vi "subscribeCommands.vi"(8 "error in (no error)":errorcluster, 11 "SAL_Listener in":refnum<class "SAL_Listener.lvclass">) -> (0 "error out":errorcluster, 3 "SAL_Listener out":refnum<class "SAL_Listener.lvclass">)   [LabVIEW 2016, in "SAL_Listener.lvclass"]
uses:
  SAL_Listener.lvclass
  SALLV_dome/SALLV_dome.lvlib
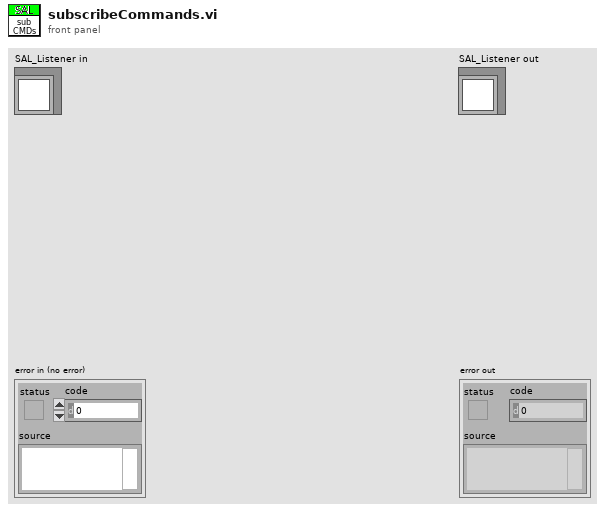
[diagram p1: front panel]
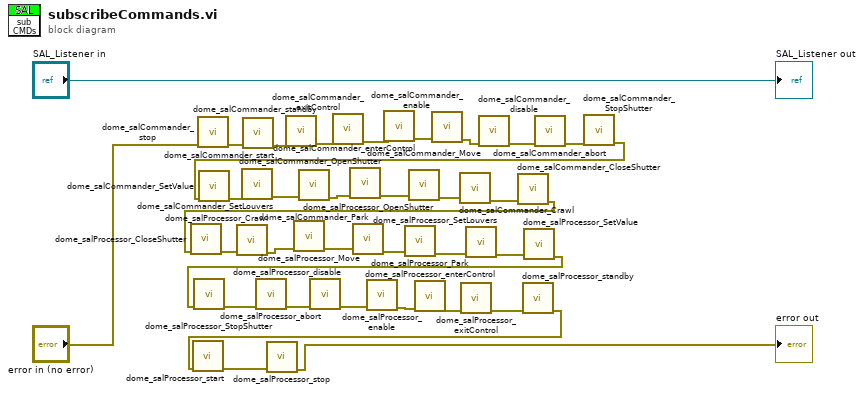
[diagram p0: block diagram]
diagram:
  n1 = call "dome_salCommander_stop.vi"("error in (no error)"="error in (no error)") -> ("error out"=w32:errorcluster)  [unwired: 9 in, 1 out]
  n2 = call "dome_salCommander_start.vi"("error in (no error)"=w32) -> ("error out"=w31:errorcluster)  [unwired: 9 in, 1 out]
  n3 = call "dome_salCommander_standby.vi"("error in (no error)"=w31) -> ("error out"=w30:errorcluster)  [unwired: 9 in, 1 out]
  n4 = call "dome_salCommander_exitControl.vi"("error in (no error)"=w30) -> ("error out"=w29:errorcluster)  [unwired: 9 in, 1 out]
  n5 = call "dome_salCommander_enterControl.vi"("error in (no error)"=w29) -> ("error out"=w28:errorcluster)  [unwired: 9 in, 1 out]
  n6 = call "dome_salCommander_enable.vi"("error in (no error)"=w28) -> ("error out"=w27:errorcluster)  [unwired: 9 in, 1 out]
  n7 = call "dome_salCommander_disable.vi"("error in (no error)"=w27) -> ("error out"=w26:errorcluster)  [unwired: 9 in, 1 out]
  n8 = call "dome_salCommander_abort.vi"("error in (no error)"=w26) -> ("error out"=w24:errorcluster)  [unwired: 9 in, 1 out]
  n9 = call "dome_salCommander_StopShutter.vi"("error in (no error)"=w24) -> ("error out"=w25:errorcluster)  [unwired: 9 in, 1 out]
  n10 = call "dome_salCommander_SetValue.vi"("error in (no error)"=w25) -> ("error out"=w23:errorcluster)  [unwired: 9 in, 1 out]
  n11 = call "dome_salCommander_SetLouvers.vi"("error in (no error)"=w23) -> ("error out"=w22:errorcluster)  [unwired: 9 in, 1 out]
  n12 = call "dome_salCommander_Park.vi"("error in (no error)"=w22) -> ("error out"=w21:errorcluster)  [unwired: 9 in, 1 out]
  n13 = call "dome_salCommander_OpenShutter.vi"("error in (no error)"=w21) -> ("error out"=w20:errorcluster)  [unwired: 9 in, 1 out]
  n14 = call "dome_salCommander_Move.vi"("error in (no error)"=w20) -> ("error out"=w19:errorcluster)  [unwired: 9 in, 1 out]
  n15 = call "dome_salCommander_Crawl.vi"("error in (no error)"=w19) -> ("error out"=w18:errorcluster)  [unwired: 9 in, 1 out]
  n16 = call "dome_salCommander_CloseShutter.vi"("error in (no error)"=w18) -> ("error out"=w17:errorcluster)  [unwired: 9 in, 1 out]
  n17 = call "dome_salProcessor_CloseShutter.vi"("error in (no error)"=w17) -> ("error out"=w16:errorcluster)  [unwired: 9 in, 1 out]
  n18 = call "dome_salProcessor_Crawl.vi"("error in (no error)"=w16) -> ("error out"=w15:errorcluster)  [unwired: 9 in, 1 out]
  n19 = call "dome_salProcessor_Move.vi"("error in (no error)"=w15) -> ("error out"=w14:errorcluster)  [unwired: 9 in, 1 out]
  n20 = call "dome_salProcessor_OpenShutter.vi"("error in (no error)"=w14) -> ("error out"=w13:errorcluster)  [unwired: 9 in, 1 out]
  n21 = call "dome_salProcessor_Park.vi"("error in (no error)"=w13) -> ("error out"=w12:errorcluster)  [unwired: 9 in, 1 out]
  n22 = call "dome_salProcessor_SetLouvers.vi"("error in (no error)"=w12) -> ("error out"=w11:errorcluster)  [unwired: 9 in, 1 out]
  n23 = call "dome_salProcessor_SetValue.vi"("error in (no error)"=w11) -> ("error out"=w10:errorcluster)  [unwired: 9 in, 1 out]
  n24 = call "dome_salProcessor_StopShutter.vi"("error in (no error)"=w10) -> ("error out"=w9:errorcluster)  [unwired: 9 in, 1 out]
  n25 = call "dome_salProcessor_abort.vi"("error in (no error)"=w9) -> ("error out"=w8:errorcluster)  [unwired: 9 in, 1 out]
  n26 = call "dome_salProcessor_disable.vi"("error in (no error)"=w8) -> ("error out"=w7:errorcluster)  [unwired: 9 in, 1 out]
  n27 = call "dome_salProcessor_enable.vi"("error in (no error)"=w7) -> ("error out"=w6:errorcluster)  [unwired: 9 in, 1 out]
  n28 = call "dome_salProcessor_enterControl.vi"("error in (no error)"=w6) -> ("error out"=w5:errorcluster)  [unwired: 9 in, 1 out]
  n29 = call "dome_salProcessor_exitControl.vi"("error in (no error)"=w5) -> ("error out"=w4:errorcluster)  [unwired: 9 in, 1 out]
  n30 = call "dome_salProcessor_standby.vi"("error in (no error)"=w4) -> ("error out"=w3:errorcluster)  [unwired: 9 in, 1 out]
  n31 = call "dome_salProcessor_start.vi"("error in (no error)"=w3) -> ("error out"=w2:errorcluster)  [unwired: 9 in, 1 out]
  n32 = call "dome_salProcessor_stop.vi"("error in (no error)"=w2) -> ("error out"=→"error out":errorcluster)  [unwired: 9 in, 1 out]
  "SAL_Listener out" <- "SAL_Listener in"
